vi "Replace column.vi"(1 "Column index":i32, 2 "Column":sgl[](array[numeric]) format="%.2e", 3 "Input array":sgl[][](array[numeric]) format="%.2e") -> (0 "Output array":sgl[][](array[numeric]) format="%.2e")   [LabVIEW 2021]
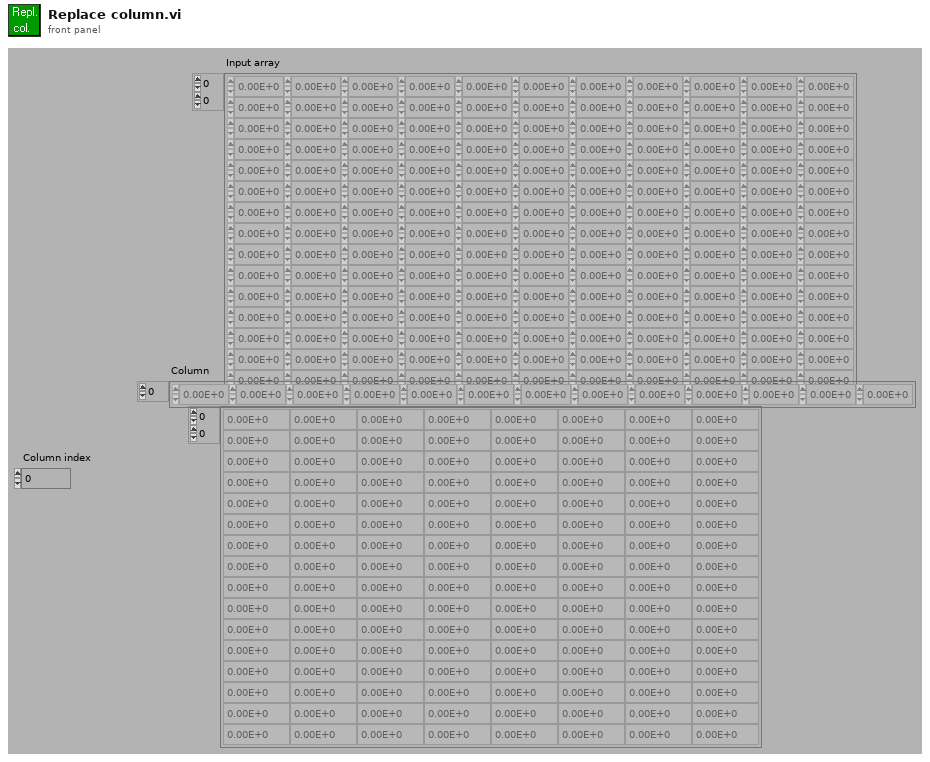
[diagram p1: front panel]
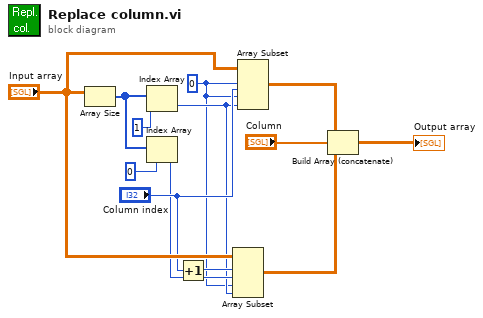
[diagram p0: block diagram]
diagram:
  w1 = 0 ("Array Index")
  n1 = Array Size(array="Input array") -> (size(s)=w12:i32[])
  n2 = Index Array(array=w12, index=1) -> (element=w3:i32)
  n3 = Index Array(array=w12, index=0) -> (element=w4:i32)
  n4 = Increment(x="Column index") -> (x+1=w5:i32)
  n5 = Array Subset(array="Input array", index (row)=w5, length (row)=w4, index (col)=w1, length (col)=w3) -> (w8:sgl[][])
  n6 = Array Subset(array="Input array", index (row)=w1, length (row)="Column index", index (col)=w1, length (col)=w3) -> (w9:sgl[][])
  n7 = Build Array (concatenate)(w9, "Column", w8) -> (→"Output array":sgl[][])
